vi "方位角位置关系.vi"(9 "输入角度":dbl format="%#_3g", 11 "基准角度":dbl format="%#_3g") -> (3 "输入角相对基准角的方位":enum16{"左侧-逆时针向", "右侧-顺时针向"}(ring))   [LabVIEW 2018]
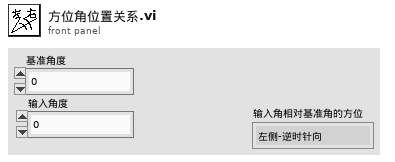
[diagram p1: front panel]
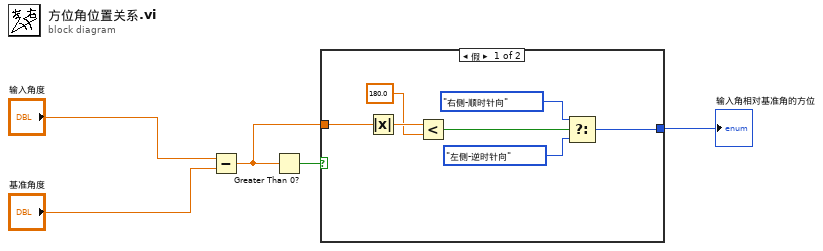
[diagram p0: block diagram]
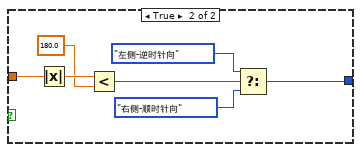
[diagram p2: hidden frame]
diagram:
  n1 = Subtract(x="输入角度", y="基准角度") -> (x-y=w5:dbl)
  n2 = Greater Than 0?(x=w5) -> (x > 0?=w4:bool)
  n3 = case shown="假" w4 {
    tunnel: w5 -> [w7 w17]
    tunnel: [w6 w13] -> w3
    frame False {
      n4 = Absolute Value(x=w7) -> (abs(x)=w12:dbl)
      n5 = Less?(x=w12, y=180.0) -> (x < y?=w10:bool)
      n6 = Select(t=enum16{"左侧-逆时针向", "右侧-顺时针向"}."右侧-顺时针向", s=w10, f=enum16{"左侧-逆时针向", "右侧-顺时针向"}."左侧-逆时针向") -> (s? t:f=w6:enum16{"左侧-逆时针向", "右侧-顺时针向"})
    }
    frame True {
      n7 = Absolute Value(x=w17) -> (abs(x)=w19:dbl)
      n8 = Less?(x=w19, y=180.0) -> (x < y?=w16:bool)
      n9 = Select(t=enum16{"左侧-逆时针向", "右侧-顺时针向"}."左侧-逆时针向", s=w16, f=enum16{"左侧-逆时针向", "右侧-顺时针向"}."右侧-顺时针向") -> (s? t:f=w13:enum16{"左侧-逆时针向", "右侧-顺时针向"})
    }
  }
  "输入角相对基准角的方位" <- w3
